vi "testConvertToKeyValuePair.vi"(8 "error in (no error)":errorcluster) -> (0 "error out":errorcluster)   [LabVIEW 2018]
doc: "Test the convertToKeyValuePair.vi."
uses:
  src/Utility/keyValuePair/convertToKeyValuePair_double.vi
  <vilib>/addons/_JKI Toolkits/Caraya/classes/Assert/Assert Equal Value_Variant.vi
  src/Utility/keyValuePair/convertToKeyValuePair_integer.vi
  src/Utility/keyValuePair/convertToKeyValuePair_boolean.vi
  src/Utility/keyValuePair/convertToKeyValuePair_string.vi
  src/Utility/keyValuePair/convertToKeyValuePair_1DArray.vi
  src/Utility/keyValuePair/convertToKeyValuePair_2DArray.vi
  <vilib>/addons/_JKI Toolkits/Caraya/classes/Test/Test.lvclass
  <vilib>/addons/_JKI Toolkits/Caraya/classes/Assert/Assert.lvclass
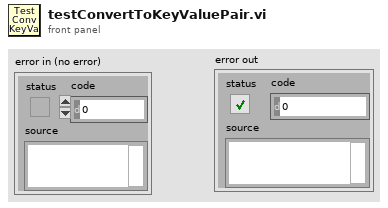
[diagram p1: front panel]
types:
  T1 = cluster{"name":string, "value":dbl[][], "precision (0)":u8}[]
  T2 = cluster{"name":string, "value":dbl[], "precision (0)":u8}[]
  T3 = cluster{"name":string, "value":dbl, "precision (0)":u8}[]
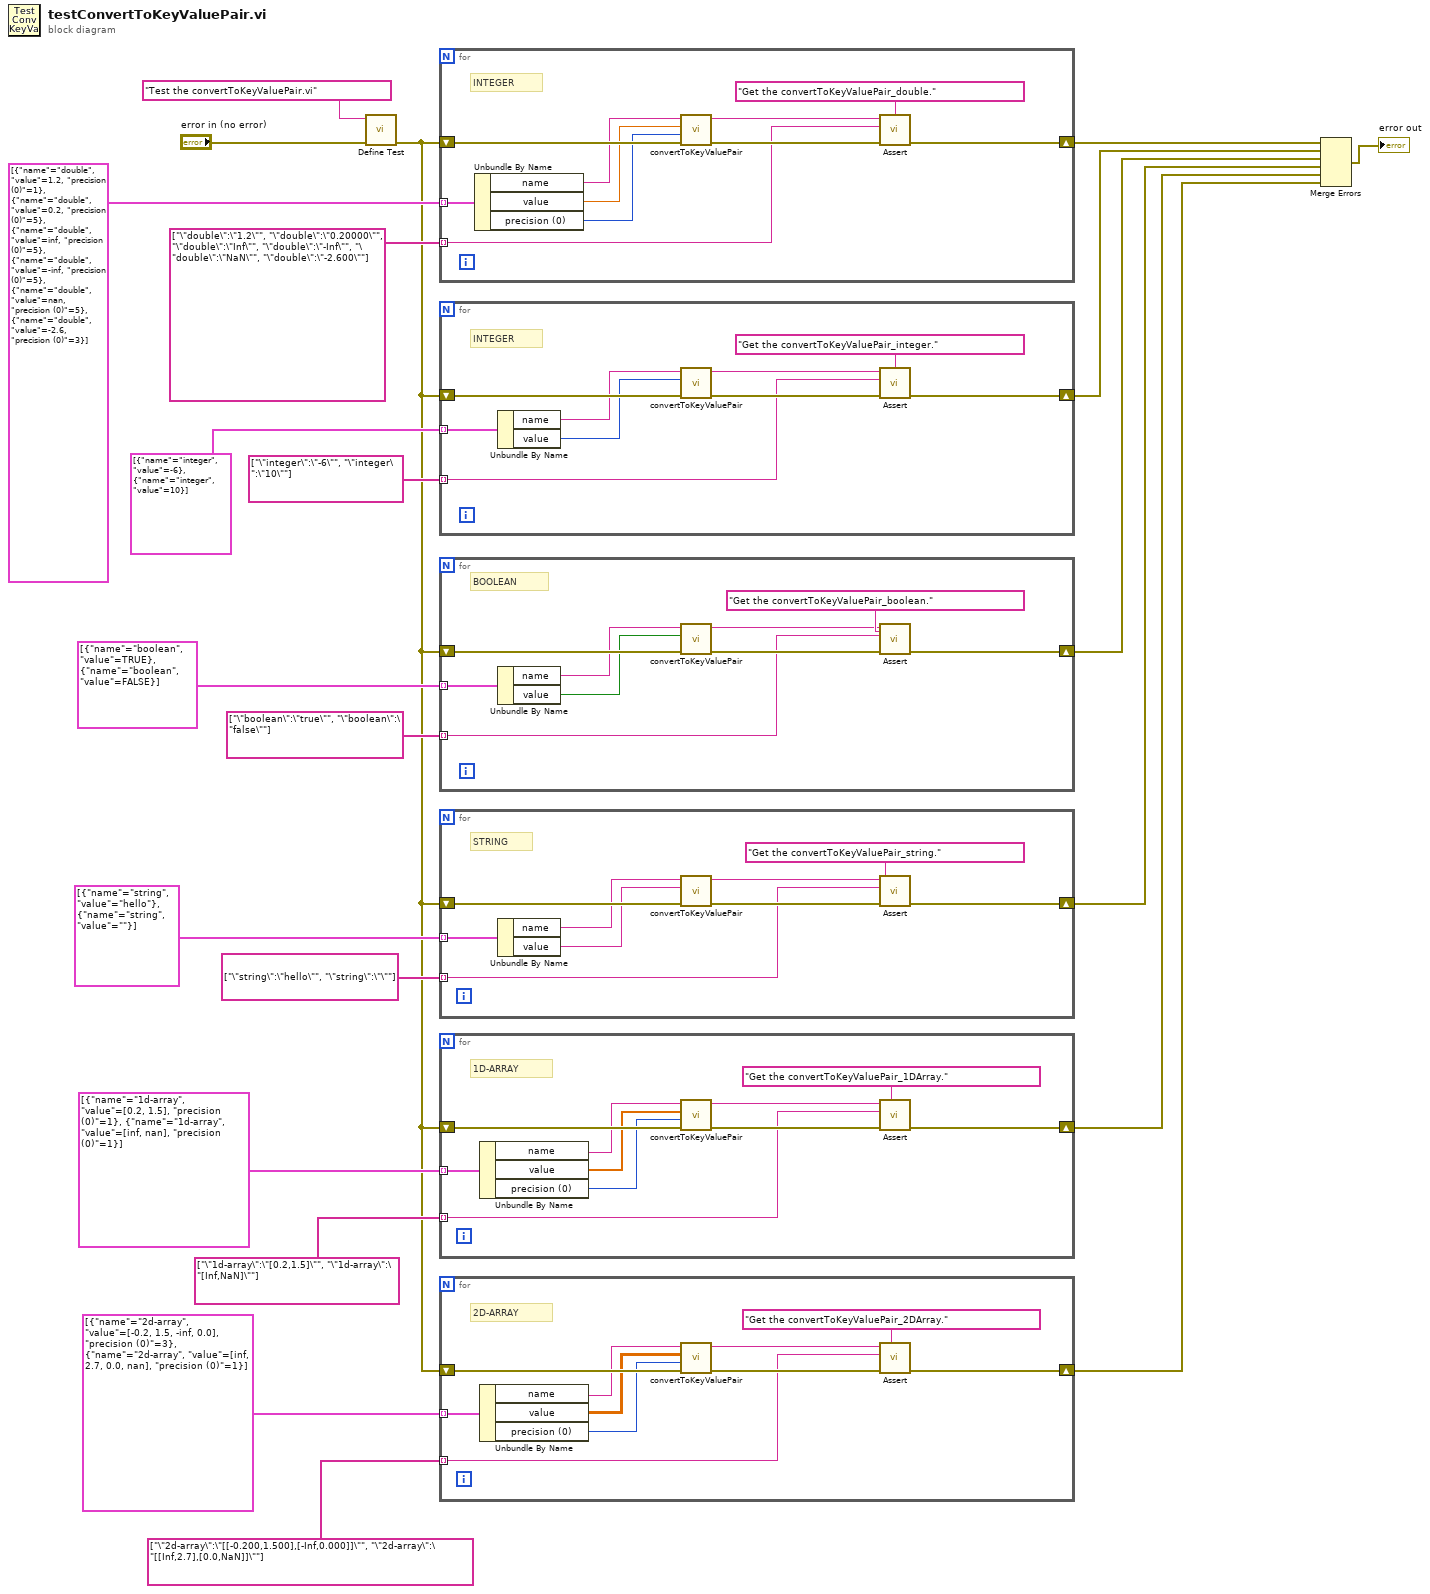
[diagram p0: block diagram]
diagram:
  n1 = call <vilib>:"Define Test.vi"("error in (no error)"="error in (no error)", "Label (VI Title)"="Test the convertToKeyValuePair.vi") -> ("error out"=w4:errorcluster)  [unwired: 9 in]
  n2 = for {
    shift-right: [w32] -> w20
    shift-left: w4 -> [w30]
    tunnel: T3 [{"name"="double", "value"=1.2, "precision (0)"=1}, {"name"="double", "value"=0.2, "precision (0)"=5}, {"name"="double", "value"=inf, "precision (0)"=5}, {"name"="double", "value"=-inf, "precision (0)"=5}, {"name"="double", "value"=nan, "precision (0)"=5}, {"name"="double", "value"=-2.6, "precision (0)"=3}] -> [w28] mode=indexing
    tunnel: string[] ["\"double\":\"1.2\"", "\"double\":\"0.20000\"", "\"double\":\"Inf\"", "\"double\":\"-Inf\"", "\"double\":\"NaN\"", "\"double\":\"-2.600\""] ("name") -> [w23] mode=indexing
    # "INTEGER"
    n3 = Unbundle By Name(w28) -> ("name"=w27:string, "value"=w26:dbl, "precision (0)"=w25:u8)
    n4 = call-poly "convertToKeyValuePair.vi"("error in (no error)"=w30, "numZeros (0)"=w25, "value"=w26, "name"=w27) -> ("error out"=w31:errorcluster, "string converted"=w24:string)  [unwired: 6 in]
    n5 = call-poly <vilib>:"Assert.vi"("Label"="Get the convertToKeyValuePair_double.", "error in (no error)"=w31, "Y"=w23, "X"=w24) -> ("error out"=w32:errorcluster)  [unwired: 7 in]
  }
  n6 = for {
    shift-right: [w41] -> w14
    shift-left: w4 -> [w39]
    tunnel: cluster{"name":string, "value":i32}[] [{"name"="integer", "value"=-6}, {"name"="integer", "value"=10}] -> [w37] mode=indexing
    tunnel: string[] ["\"integer\":\"-6\"", "\"integer\":\"10\""] -> [w33] mode=indexing
    # "INTEGER"
    n7 = Unbundle By Name(w37) -> ("name"=w36:string, "value"=w35:i32)
    n8 = call-poly "convertToKeyValuePair.vi"("error in (no error)"=w39, "value"=w35, "name"=w36) -> ("error out"=w40:errorcluster, "string converted"=w34:string)  [unwired: 7 in]
    n9 = call-poly <vilib>:"Assert.vi"("Label"="Get the convertToKeyValuePair_integer.", "error in (no error)"=w40, "Y"=w33, "X"=w34) -> ("error out"=w41:errorcluster)  [unwired: 7 in]
  }
  n10 = for {
    shift-right: [w50] -> w11
    shift-left: w4 -> [w48]
    tunnel: cluster{"name":string, "value":bool}[] [{"name"="boolean", "value"=TRUE}, {"name"="boolean", "value"=FALSE}] -> [w46] mode=indexing
    tunnel: string[] ["\"boolean\":\"true\"", "\"boolean\":\"false\""] -> [w42] mode=indexing
    # "BOOLEAN"
    n11 = Unbundle By Name(w46) -> ("name"=w45:string, "value"=w44:bool)
    n12 = call-poly "convertToKeyValuePair.vi"("error in (no error)"=w48, "value"=w44, "name"=w45) -> ("error out"=w49:errorcluster, "string converted"=w43:string)  [unwired: 7 in]
    n13 = call-poly <vilib>:"Assert.vi"("Label"="Get the convertToKeyValuePair_boolean.", "error in (no error)"=w49, "Y"=w42, "X"=w43) -> ("error out"=w50:errorcluster)  [unwired: 7 in]
  }
  n14 = for {
    shift-right: [w59] -> w8
    shift-left: w4 -> [w57]
    tunnel: cluster{"name":string, "value":string}[] [{"name"="string", "value"="hello"}, {"name"="string", "value"=""}] -> [w54] mode=indexing
    tunnel: string[] ["\"string\":\"hello\"", "\"string\":\"\""] -> [w51] mode=indexing
    # "STRING"
    n15 = Unbundle By Name(w54) -> ("name"=w53:string, "value"=w52:string)
    n16 = call-poly "convertToKeyValuePair.vi"("error in (no error)"=w57, "value"=w52, "name"=w53) -> ("error out"=w58:errorcluster, "string converted"=w55:string)  [unwired: 7 in]
    n17 = call-poly <vilib>:"Assert.vi"("Label"="Get the convertToKeyValuePair_string.", "error in (no error)"=w58, "Y"=w51, "X"=w55) -> ("error out"=w59:errorcluster)  [unwired: 7 in]
  }
  n18 = for {
    shift-right: [w69] -> w5
    shift-left: w4 -> [w67]
    tunnel: string[] ["\"1d-array\":\"[0.2,1.5]\"", "\"1d-array\":\"[Inf,NaN]\""] -> [w64] mode=indexing
    tunnel: T2 [{"name"="1d-array", "value"=[0.2, 1.5], "precision (0)"=1}, {"name"="1d-array", "value"=[inf, nan], "precision (0)"=1}] -> [w63] mode=indexing
    # "1D-ARRAY"
    n19 = Unbundle By Name(w63) -> ("name"=w62:string, "value"=w61:dbl[], "precision (0)"=w60:u8)
    n20 = call-poly "convertToKeyValuePair.vi"("error in (no error)"=w67, "presicion (0)"=w60, "value"=w61, "name"=w62) -> ("error out"=w68:errorcluster, "string converted"=w65:string)  [unwired: 6 in]
    n21 = call-poly <vilib>:"Assert.vi"("Label"="Get the convertToKeyValuePair_1DArray.", "error in (no error)"=w68, "Y"=w64, "X"=w65) -> ("error out"=w69:errorcluster)  [unwired: 7 in]
  }
  n22 = for {
    shift-right: [w79] -> w1
    shift-left: w4 -> [w77]
    tunnel: string[] ["\"2d-array\":\"[[-0.200,1.500],[-Inf,0.000]]\"", "\"2d-array\":\"[[Inf,2.7],[0.0,NaN]]\""] -> [w74] mode=indexing
    tunnel: T1 [{"name"="2d-array", "value"=[[-0.2, 1.5], [-inf, 0.0]], "precision (0)"=3}, {"name"="2d-array", "value"=[[inf, 2.7], [0.0, nan]], "precision (0)"=1}] -> [w73] mode=indexing
    # "2D-ARRAY"
    n23 = Unbundle By Name(w73) -> ("name"=w72:string, "value"=w71:dbl[][], "precision (0)"=w70:u8)
    n24 = call-poly "convertToKeyValuePair.vi"("error in (no error)"=w77, "presicion (0)"=w70, "value"=w71, "name"=w72) -> ("error out"=w78:errorcluster, "string converted"=w75:string)  [unwired: 6 in]
    n25 = call-poly <vilib>:"Assert.vi"("Label"="Get the convertToKeyValuePair_2DArray.", "error in (no error)"=w78, "Y"=w74, "X"=w75) -> ("error out"=w79:errorcluster)  [unwired: 7 in]
  }
  n26 = Merge Errors(w20, w14, w11, w8, w5, w1) -> (→"error out":errorcluster)
